vi "cumulate cpx in string (host).vi"(11 "Data":u64[](array[numeric])) -> (3 "String":string)   [LabVIEW 2020]
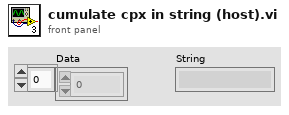
[diagram p1: front panel]
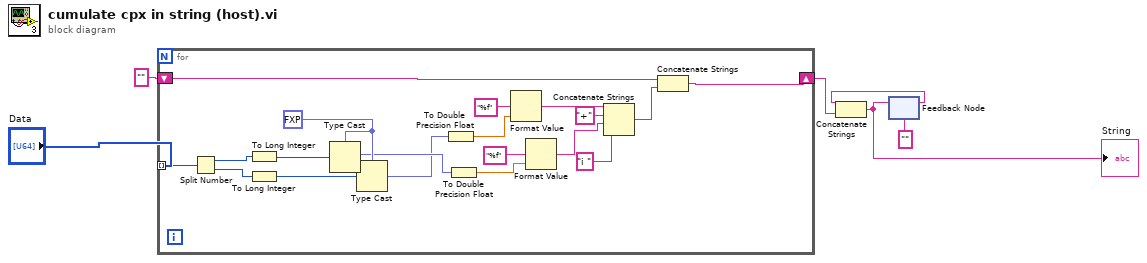
[diagram p0: block diagram]
diagram:
  n1 = for {
    tunnel: "Data" -> [w12] mode=indexing
    shift-right: [w7] -> w2
    shift-left: "" -> [w9]
    w22 = fxp<+/-,32,11> 0.0 ("Number of Elements")
    n2 = Split Number(x=w12) -> (hi(x)=w25:u32, lo(x)=w24:u32)
    n3 = To Long Integer(number=w25) -> (32bit integer=w23:i32)
    n4 = To Long Integer(number=w24) -> (32bit integer=w11:i32)
    n5 = Type Cast(type=w22, x=w23) -> (*(type *) &x=w20:fxp<+/-,32,11>)
    n6 = Type Cast(type=w22, x=w11) -> (*(type *) &x=w10:fxp<+/-,32,11>)
    n7 = To Double Precision Float(number=w10) -> (double precision float=w19:dbl)
    n8 = To Double Precision Float(number=w20) -> (double precision float=w17:dbl)
    n9 = Format Value(format string="%f", value (0)=w19) -> (output string=w16:string)  [unwired: 1 in]
    n10 = Format Value(format string="%f", value (0)=w17) -> (output string=w14:string)  [unwired: 1 in]
    n11 = Concatenate Strings(w16, "+" ("string"), w14, "i " ("string")) -> (w8:string)
    n12 = Concatenate Strings(w9, w8) -> (w7:string)
  }
  n13 = feedback #1("" ("output string")) -> (w5:string)
  n14 = Concatenate Strings(w5, w2) -> (w4:string)
  "String" <- w4
  n15 = feedback-in #1(w4) -> ()
